vi "Subsystem Sequencer Cancel.vi"   [LabVIEW 2017]
doc: "This template has a parameter to control whether it waits for the command to complete or not. This is useful for operations that have a timed duration or a sensor-based duration. \n\nBe sure to right-click and select New from Template and save with a new command name."
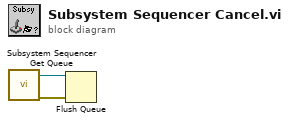
[diagram p0: block diagram]
diagram:
  n1 = call "Subsystem Sequencer Get Queue.vi"() -> ("error out"=w2:errorcluster, "queue out"=w1:refnum<queue>)  [unwired: 10 in]
  n2 = Flush Queue(queue=w1, error in (no error)=w2) -> ()  [unwired: 3 out]
